vi "Parse.vi"(8 "error in (no error)":errorcluster, 10 "File to Parse":path, 11 "File Parsing Interface in":refnum<class "File Parsing Interface.lvclass">) -> (0 "error out":errorcluster, 2 "Measurements Out":T1[](array[typedef]), 3 "File Parsing Interface out":refnum<class "File Parsing Interface.lvclass">)   [LabVIEW 2018, in "File Parsing Interface.lvlib" / "File Parsing Interface.lvclass"]
uses:
  File Parsing Interface.lvclass
  Controls/Parsed Measurement.ctl
  Plugins/Measurement Data.lvlibp/Measurement Data.lvclass
  File Parsing Interface.lvclass/File Parsing Interface.ctl
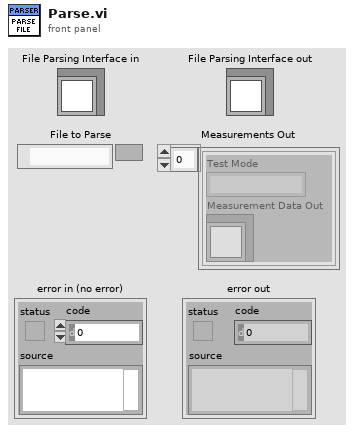
[diagram p1: front panel]
types:
  T1 = typedef "File Parsing Interface.lvlib/File Parsing Interface.lvclass/Parsed Measurement.ctl" = cluster{"Test Mode":string, "Measurement Data Out":refnum<class "Measurement Data.lvclass">}
  T2 = cluster{"Test Mode":string, "Measurement Data Out":refnum<class "Measurement Data.lvclass">}[]
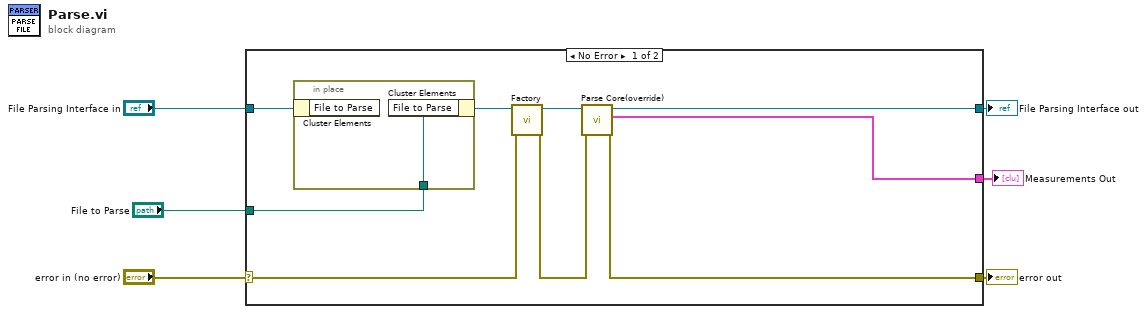
[diagram p0: block diagram]
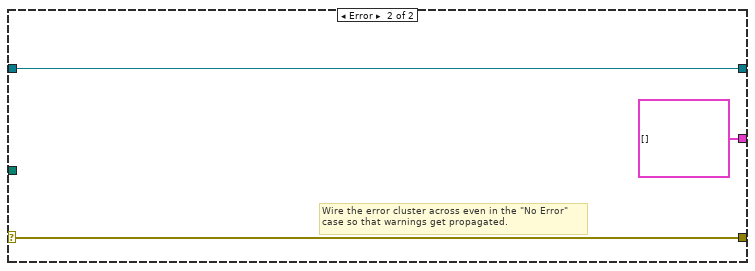
[diagram p2: hidden frame]
diagram:
  n1 = case shown="No Error" "error in (no error)" {
    selector: "error in (no error)" -> [w15 w19]
    tunnel: [w13 w19] -> w5
    tunnel: [w11 w18] -> w3
    tunnel: "File Parsing Interface in" -> [w10 w18]
    tunnel: "File to Parse" -> [w8 _]
    tunnel: [w7 T2 [] ("Measurements Out")] -> w1
    frame No Error {
      n2 = in-place {
        in-place-border: w8 -> [w16]
        n3 = in-place-cluster #1(w10) -> ()  [unwired: 1 out]
        n4 = in-place-cluster #1("File to Parse"=w16) -> (w9:refnum<class "File Parsing Interface.lvclass">)
      }
      n5 = call-dynamic "Factory.vi"("error in (no error)"=w15, "File Parsing Interface in"=w9) -> ("error out"=w14:errorcluster, "File Parsing Interface out"=w12:refnum<class "File Parsing Interface.lvclass">)  [unwired: 8 in]
      n6 = call-dynamic "Parse Core(override).vi"("error in (no error)"=w14, "File Parsing Interface in"=w12) -> ("error out"=w13:errorcluster, "Measurements Out"=w7:T1[], "File Parsing Interface out"=w11:refnum<class "File Parsing Interface.lvclass">)  [unwired: 7 in]
    }
    frame Error {
      # "Wire the error cluster across even in the \"No Error\"\ncase so that warnings get propagated."
    }
  }
  "error out" <- w5
  "File Parsing Interface out" <- w3
  "Measurements Out" <- w1
